vi "destroy.vi"(0 "data_simple_pipeline in":refnum<class "data_simple_pipeline.lvclass">, 11 "error in (no error)":errorcluster) -> (4 "data_simple_pipeline out":refnum<class "data_simple_pipeline.lvclass">, 15 "error out":errorcluster)   [LabVIEW 2020, in "data_simple_pipeline.lvclass"]
uses:
  data_simple_pipeline.lvclass
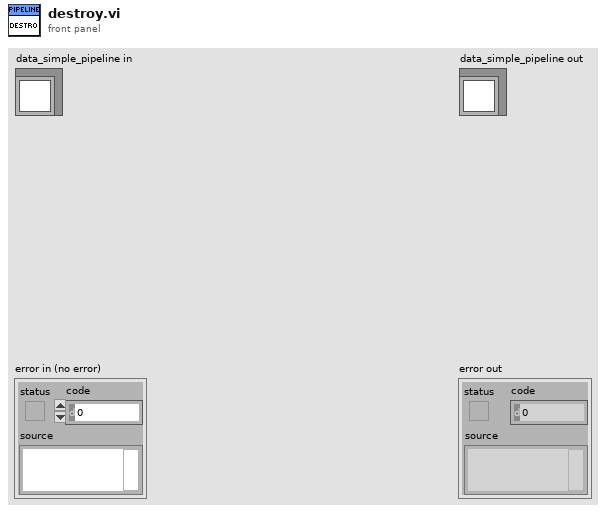
[diagram p1: front panel]
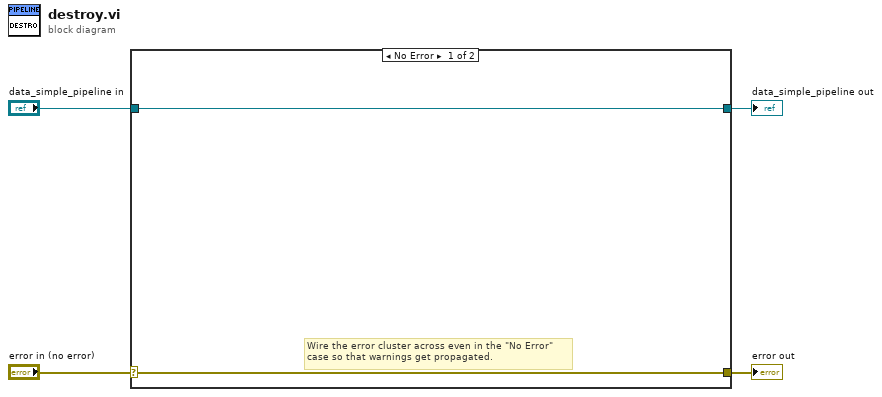
[diagram p0: block diagram]
diagram:
  n1 = case shown="No Error" "error in (no error)" {
    selector: "error in (no error)" -> [w5 w8]
    tunnel: [w5 w8] -> w3
    tunnel: [w6 w7] -> w1
    tunnel: "data_simple_pipeline in" -> [w6 w7]
    frame No Error {
      # "Wire the error cluster across even in the \"No Error\"\ncase so that warnings get propagated."
    }
    frame Error {
    }
  }
  "error out" <- w3
  "data_simple_pipeline out" <- w1
